vi "Albert_SQL_101.vi"(7 "表名":string, 8 "error in (no error)":errorcluster, 10 "查询语句":string, 11 "connection reference":T1) -> (0 "error out":errorcluster, 2 "数据":string[][](array[string]), 3 "connection reference out":T1)   [LabVIEW 2018]
uses:
  <vilib>/addons/database/Connection.llb/Conn ObjectReference.ctl
  <vilib>/addons/database/Connection.llb/Conn Execute.vi
  <vilib>/addons/database/Recordset.llb/Rec Fetch Recordset Data (R).vi
  <vilib>/addons/database/Recordset.llb/Rec Destroy - Connection.vi
  <vilib>/addons/database/NI_Database_API.lvlib
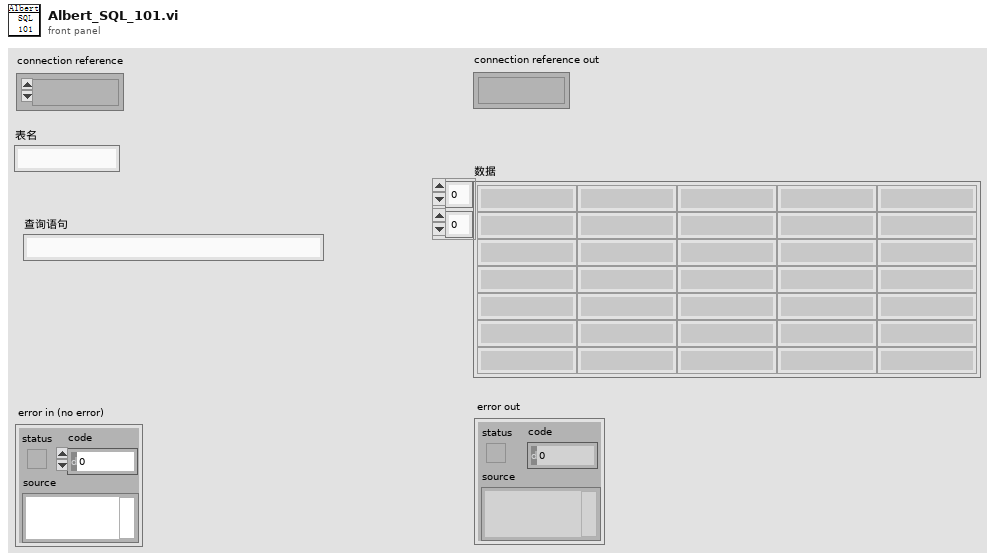
[diagram p1: front panel]
types:
  T1 = typedef "NI_Database_API.lvlib/Conn ObjectReference.ctl" = refnum<k1>
  T2 = typedef "NI_Database_API.lvlib/Rec ObjectReference.ctl" = refnum<k1>
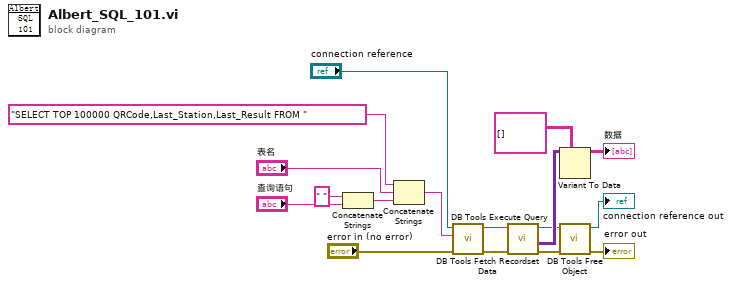
[diagram p0: block diagram]
diagram:
  n1 = Concatenate Strings(" ", "查询语句") -> (w1:string)
  n2 = Concatenate Strings("SELECT TOP 100000 QRCode,Last_Station,Last_Result FROM " ("字符串"), "表名", w1) -> (w10:string)
  n3 = call-poly <vilib>:"DB Tools Execute Query.vi"("error in (no error)"="error in (no error)", "SQL query"=w10, "connection reference"="connection reference") -> ("error out"=w7:errorcluster, "recordset reference"=w11:T2)  [unwired: 5 in]
  n4 = call-poly <vilib>:"DB Tools Fetch Recordset Data.vi"("error in (no error)"=w7, "recordset reference"=w11) -> ("error out"=w6:errorcluster, "recordset data"=w14:variant[][], "recordset reference out"=w13:T2)  [unwired: 3 in]
  n5 = Variant To Data(type=string[][] [], Variant=w14) -> (data=→"数据":string[][])  [unwired: 1 in, 1 out]
  n6 = call-poly <vilib>:"DB Tools Free Object.vi"("error in (no error)"=w6, "recordset reference"=w13) -> ("error out"=→"error out":errorcluster, "connection reference"=→"connection reference out":T1)  [unwired: 8 in]
